vi "S706 Parameter senden.vi"(8 "Fehler (Eingang)":errorcluster, 10 "SDO object in":refnum<k20>, 11 "Dateipfad (Dialog verwenden)":path) -> (0 "error out":errorcluster)   [LabVIEW 2014]
uses:
  <vilib>/CANopenLib/CANOPEN.llb/CANopen SDO Write [STR].vi
  <vilib>/CANopenLib/CANOPEN.llb/CANopen SDO Write [I32].vi
  <vilib>/regexp/Match Regular Expression.xnode
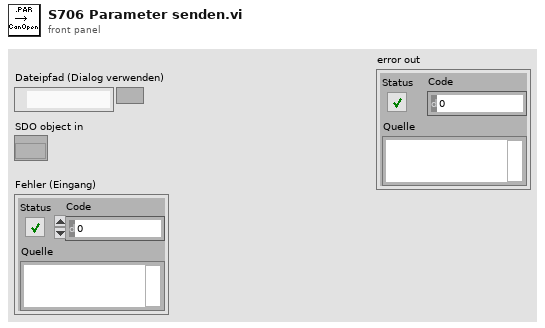
[diagram p1: front panel]
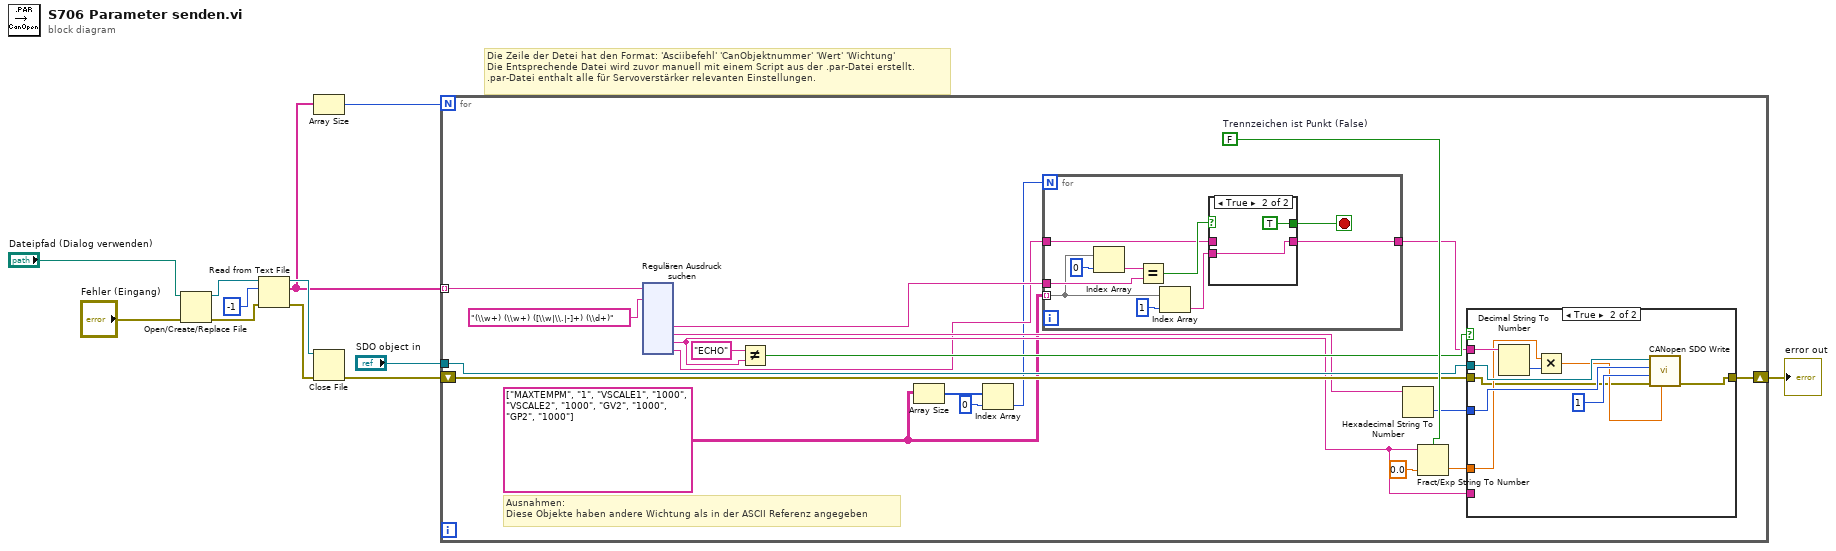
[diagram p0: block diagram]
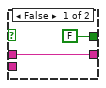
[diagram p2: hidden frame]
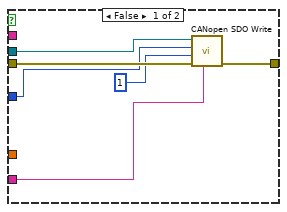
[diagram p3: hidden frame]
diagram:
  # "Die Zeile der Detei hat den Format: 'Asciibefehl' 'CanObjektnummer' 'Wert' 'Wichtung'\nDie Entsprechende Datei wird zuvor manuell mit einem Script aus der .par-Datei erstellt. \n.par-Datei enthalt alle für Servoverstärker relevanten Einstellungen."
  n1 = Open/Create/Replace File(file path (use dialog)="Dateipfad (Dialog verwenden)", error in="Fehler (Eingang)") -> (refnum out=w12:refnum<file>, error out=w2:errorcluster)  [unwired: 4 in, 1 out]
  n2 = Read from Text File(file (use dialog)=w12, count=-1 ("Anzahl"), error in=w2) -> (refnum out=w10:refnum<file>, text=w7:string[], error out=w9:errorcluster)  [unwired: 1 in, 1 out]
  n3 = Array Size(array=w7) -> (size(s)=w8:i32)
  n4 = Close File(refnum=w10, error in=w9) -> (error out=w5:errorcluster)  [unwired: 1 out]
  n5 = for {
    N: w8 -> [_]
    tunnel: w7 -> [w31] mode=indexing
    tunnel: "SDO object in" -> [w26]
    shift-right: [w28] -> w4
    shift-left: w5 -> [w24]
    w16 = string[][] [["MAXTEMPM", "1"], ["VSCALE1", "1000"], ["VSCALE2", "1000"], ["GV2", "1000"], ["GP2", "1000"]]
    w30 = FALSE  # Trennzeichen ist Punkt (False)
    # "Ausnahmen:\nDiese Objekte haben andere Wichtung als in der ASCII Referenz angegeben"
    n6 = xnode "Regulären Ausdruck suchen"("Eingangs-String"=w31, "Regulärer Ausdruck"="(\\w+) (\\w+) ([\\w|\\.|-]+) (\\d+)") -> ("Teilweise Übereinstimmung 1"=w19:string, "Teilweise Übereinstimmung 2"=w20:string, "Teilweise Übereinstimmung 3"=w21:string, "Teilweise Übereinstimmung 4"=w18:string)  [unwired: 4 in, 5 out]
    n7 = Not Equal?(x="ECHO", y=w21) -> (x != y?=w22:bool)
    n8 = Array Size(array=w16) -> (size(s)=w15:i32[])
    n9 = Index Array(array=w15, index=0 ("Index")) -> (element=w13:i32)
    n10 = for {
      N: w13 -> [_]
      tunnel: w16 -> [w35] mode=indexing
      tunnel: w19 -> [w42]
      tunnel: w18 -> [w39]
      tunnel: [w38] -> w17
      stop <- w41 stop-if-true
      n11 = Index Array(array=w35, index=0 ("Index")) -> (element=w36:string)
      n12 = Equal?(x=w36, y=w42) -> (x = y?=w40:bool)
      n13 = Index Array(array=w35, index=1 ("Index")) -> (element=w33:string)
      n14 = case shown="True" w40 {
        tunnel: [FALSE TRUE] -> w41
        tunnel: w39 -> [w43 _]
        tunnel: [w43 w45] -> w38
        tunnel: w33 -> [_ w45]
        frame False {
        }
        frame True {
        }
      }
    }
    n15 = Hexadecimal String To Number(string=w20) -> (number=w27:u32)  [unwired: 2 in, 1 out]
    n16 = Fract/Exp String To Number(use system decimal point (T)=w30, string=w21, default (0 dbl)=0.0 ("Standard (0 DBL)")) -> (number=w25:dbl)  [unwired: 1 in, 1 out]
    n17 = case shown="True" w22 {
      tunnel: [w52 w60] -> w28
      tunnel: w27 -> [w49 w59]
      tunnel: w26 -> [w50 w58]
      tunnel: w17 -> [_ w55]
      tunnel: w25 -> [_ w54]
      tunnel: w24 -> [w51 w53]
      tunnel: w21 -> [w47 _]
      frame False {
        n18 = call-poly <vilib>:"CANopen SDO Write.vi"("string data"=w47, "error in (no error)"=w51, "object sub-index (0)"=u8 1, "object index"=w49, "SDO object in"=w50) -> ("error out"=w52:errorcluster)  [unwired: 4 in, 2 out]
      }
      frame True {
        n19 = Decimal String To Number(string=w55) -> (number=w56:i32)  [unwired: 2 in, 1 out]
        n20 = Multiply(x=w54, y=w56) -> (x*y=w57:dbl)
        n21 = call-poly <vilib>:"CANopen SDO Write.vi"("I32 data"=w57, "error in (no error)"=w53, "object sub-index (0)"=u8 1, "object index"=w59, "SDO object in"=w58) -> ("error out"=w60:errorcluster)  [unwired: 4 in, 2 out]
      }
    }
  }
  "error out" <- w4
